vi "Main.vi"() -> ()   [LabVIEW 2018]
uses:
  F:/Program Files (x86)/National Instruments/LabVIEW 2018/examples/Instrument IO/Serial/support/Serial - Settings.ctl
panel:
  out "Response":string
  in  "Command":string="*IDN?"
  in  "쓰기?":bool
  in  "Serial Settings":T1={"baud rate"=9600, "data bits"=8, "parity"=enum."None", "stop bits"=10, "flow control"=0} {"flow control" items=["None"=0, "XON/XOFF"=1, "RTS/CTS"=2, "DTR/DSR"=4]; "stop bits" items=["1.0"=10, "1.5"=15, "2.0"=20]; "data bits" min=5 max=8 step=1; "baud rate" items=["75"=75, "110"=110, "134"=134, "150"=150, "300"=300, "600"=600, "1200"=1200, "1800"=1800, "2400"=2400, "4800"=4800, "7200"=7200, "9600"=9600, "14400"=14400, "19200"=19200, "28800"=28800, "38400"=38400, "56000"=56000, "57600"=57600, "115200"=115200, "128000"=128000, "230400"=230400]}
  in  "VISA resource name":refnum<visa-resource-name>="COM1"
  in  "정지":bool
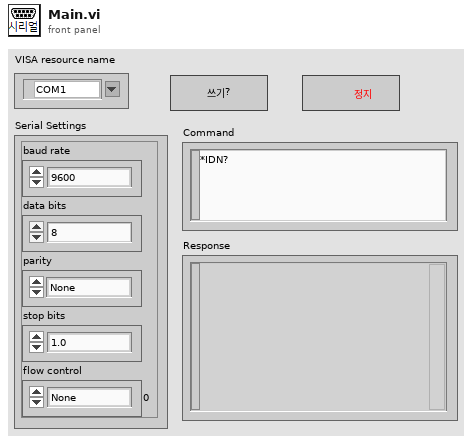
[diagram p1: front panel]
types:
  T1 = typedef "Serial - Settings.ctl" = cluster{"baud rate":u32, "data bits":u16, "parity":enum16{"None", "Odd", "Even", "Mark", "Space"}, "stop bits":u16, "flow control":u16}
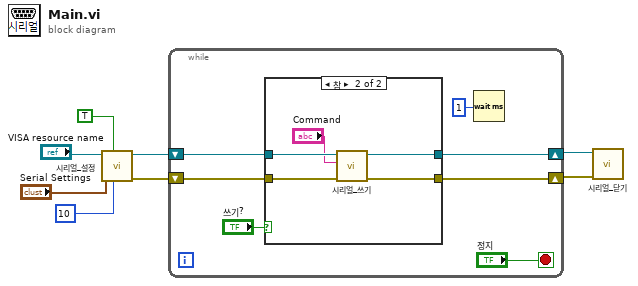
[diagram p0: block diagram]
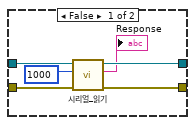
[diagram p2: hidden frame]
diagram:
  n1 = call "시리얼_설정.vi"("Termination Character"=u8 10, "End Read on Termination Character?"=TRUE, "Serial Settings"="Serial Settings", "VISA resource name"="VISA resource name") -> ("Error Out"=w3:errorcluster, "VISA resource name out"=w4:refnum<visa-resource-name>)  [unwired: 6 in]
  n2 = while {
    shift-right: [w11] -> w2
    shift-left: w4 -> [w13]
    shift-right: [w10] -> w1
    shift-left: w3 -> [w12]
    stop <- "정지" stop-if-true
    n3 = case shown="참" "쓰기?" {
      tunnel: w13 -> [w21 w26]
      tunnel: w12 -> [w20 w25]
      tunnel: [w18 w23] -> w11
      tunnel: [w19 w22] -> w10
      frame False {
        n4 = call "시리얼_읽기.vi"("Error In"=w20, "Read Count"=u32 1000, "VISA 리소스 이름"=w21) -> ("Error Out"=w19:errorcluster, "Response"=→"Response":string, "VISA 리소스 이름 출력"=w18:refnum<visa-resource-name>)  [unwired: 6 in]
      }
      frame True {
        n5 = call "시리얼_쓰기.vi"("Error In"=w25, "Command"="Command", "VISA 리소스 이름"=w26) -> ("Error Out"=w22:errorcluster, "VISA 리소스 이름 출력"=w23:refnum<visa-resource-name>)  [unwired: 7 in]
      }
    }
    n6 = Wait (ms)(milliseconds to wait=u32 1 ("ms 타이머 값")) -> ()  [unwired: 1 out]
  }
  n7 = call "시리얼_닫기.vi"("Error In"=w1, "VISA 리소스 이름"=w2) -> ()  [unwired: 9 in, 1 out]
